vi "Initial_Lootkup Table - Sin Acq Point FXP.vi"(8 "Effecte Pixel/Line":dbl=512.0, 9 "Fill Fraction":dbl=0.85, 10 "Scanning Speed":dbl=2000.0, 11 "Sample Rate":dbl=120000000.0 format="%#_6p") -> (2 "Init Data Out U16":u16[](array[numeric]), 3 "Init Data Out":fxp<+,16,0>[](array[numeric]) format="%.16g")   [LabVIEW 2015]
panel:
  out "Total Pixel/Line":dbl
  out "Average Per Pixel Dis.":dbl[][](graph)
  out "Total Average Per Pixel":dbl[](array[numeric])
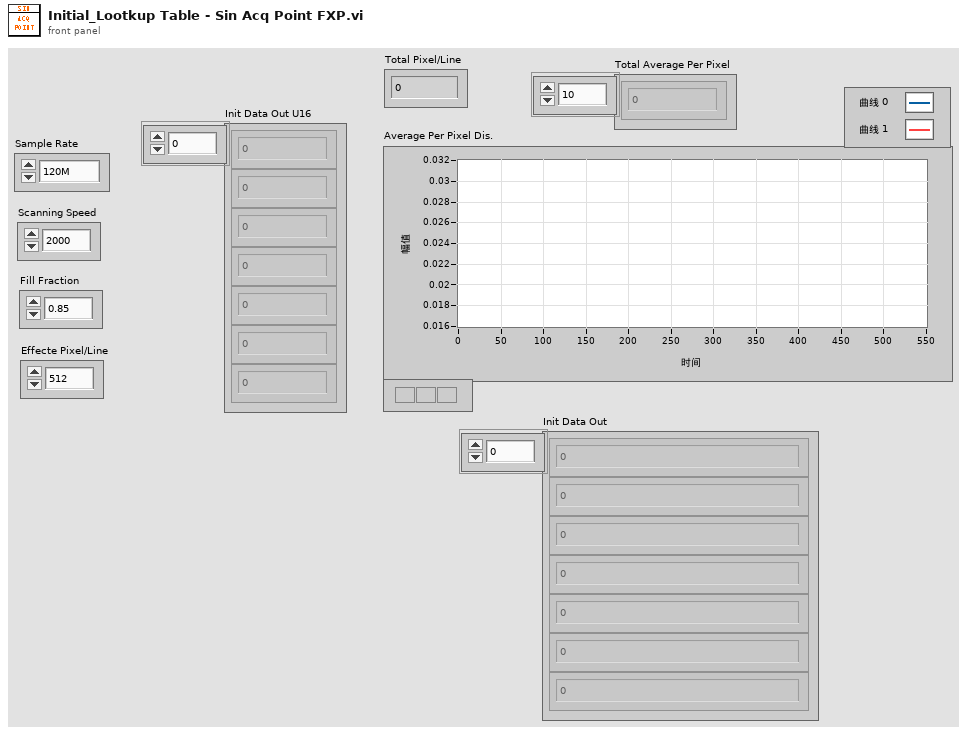
[diagram p1: front panel]
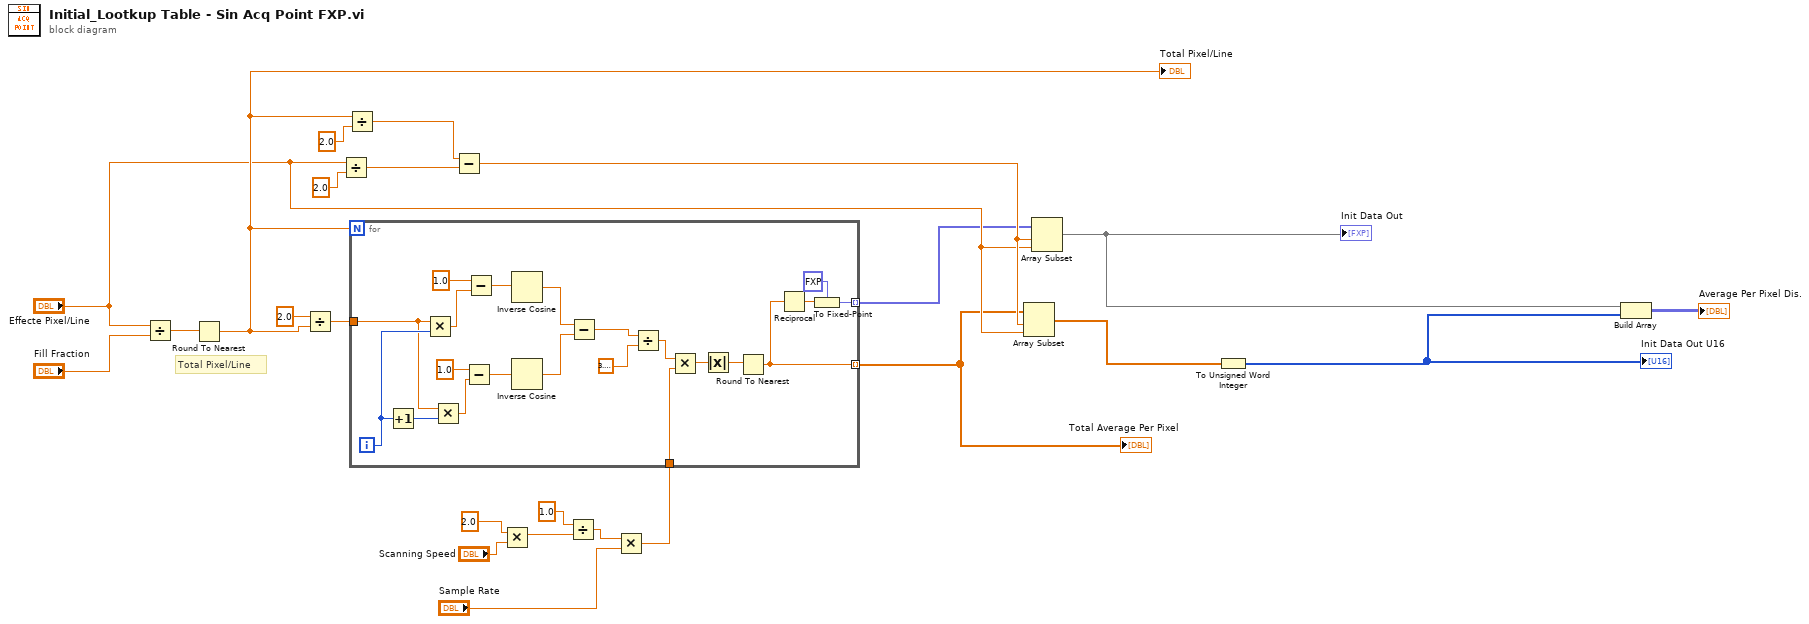
[diagram p0: block diagram]
diagram:
  # "Total Pixel/Line"
  n1 = Divide(x="Effecte Pixel/Line", y="Fill Fraction") -> (x/y=w23:dbl)
  n2 = Round To Nearest(number=w23) -> (nearest integer value=w13:dbl)
  "Total Pixel/Line" <- w13
  n3 = Divide(x=2.0, y=w13) -> (x/y=w21:dbl)
  n4 = Divide(x="Effecte Pixel/Line", y=2.0) -> (x/y=w9:dbl)
  n5 = Divide(x=w13, y=2.0) -> (x/y=w11:dbl)
  n6 = Subtract(x=w11, y=w9) -> (x-y=w6:dbl)
  n7 = Multiply(x=2.0, y="Scanning Speed") -> (x*y=w16:dbl)
  n8 = Divide(x=1.0, y=w16) -> (x/y=w15:dbl)
  n9 = Multiply(x=w15, y="Sample Rate") -> (x*y=w19:dbl)
  n10 = for {
    N: w13 -> [_]
    tunnel: w21 -> [w36]
    tunnel: w19 -> [w31]
    tunnel: [w29] -> w3 mode=indexing
    tunnel: [w26] -> w2 mode=indexing
    i -> [w39]
    n11 = Increment(x=w39) -> (x+1=w38:i32)
    n12 = Multiply(x=w36, y=w39) -> (x*y=w41:dbl)
    n13 = Multiply(x=w36, y=w38) -> (x*y=w37:dbl)
    n14 = Subtract(x=1.0, y=w37) -> (x-y=w35:dbl)
    n15 = Subtract(x=1.0, y=w41) -> (x-y=w42:dbl)
    n16 = Inverse Cosine(1:w42) -> (0:w45:dbl)
    n17 = Inverse Cosine(1:w35) -> (0:w44:dbl)
    n18 = Subtract(x=w45, y=w44) -> (x-y=w34:dbl)
    n19 = Divide(x=w34, y=3.141592653589793) -> (x/y=w32:dbl)
    n20 = Multiply(x=w32, y=w31) -> (x*y=w28:dbl)
    n21 = Absolute Value(x=w28) -> (abs(x)=w27:dbl)
    n22 = Round To Nearest(number=w27) -> (nearest integer value=w26:dbl)
    n23 = Reciprocal(x=w26) -> (1/x=w30:dbl)
    n24 = To Fixed-Point(fixed-point type=fxp<+,16,0> 0.0 ("Y Amplitude"), number=w30) -> (fixed-point=w29:fxp<+,16,0>)
  }
  "Total Average Per Pixel" <- w2
  n25 = Array Subset(array=w2, index=w6, length="Effecte Pixel/Line") -> (w4:dbl[])
  n26 = Array Subset(array=w3, index=w6, length="Effecte Pixel/Line") -> (w1:fxp<+,16,0>[])
  "Init Data Out" <- w1
  n27 = To Unsigned Word Integer(number=w4) -> (unsigned 16bit integer=w7:u16[])
  "Init Data Out U16" <- w7
  n28 = Build Array(w1, w7) -> (→"Average Per Pixel Dis.":fxp<+,32,16>[][])
